vi "Get Param Info.vi"(8 "error in (no error)":errorcluster, 11 "paramID":i32) -> (0 "error out":errorcluster, 1 "paramMin out":dbl, 2 "paramReadOnly out":i32, 3 "function return":i32, 4 "paramMax out":dbl, 5 "paramAvailable out":i32, 6 "paramDefault out":dbl, 7 "paramType out":i32)   [LabVIEW 2020, in "MPH16.lvlib"]
doc: "long GetParamInfo(const long paramID, long &paramType, long &paramAvailable, long &paramReadOnly, double &paramMin, double &paramMax, double &paramDefault);"
uses:
  MPH16.lvlib
  ThorPinholeStepper.dll
panel:
  in  "paramDefault":dbl
  in  "paramMax":dbl
  in  "paramMin":dbl
  in  "paramReadOnly":i32
  in  "paramAvailable":i32
  in  "paramType":i32
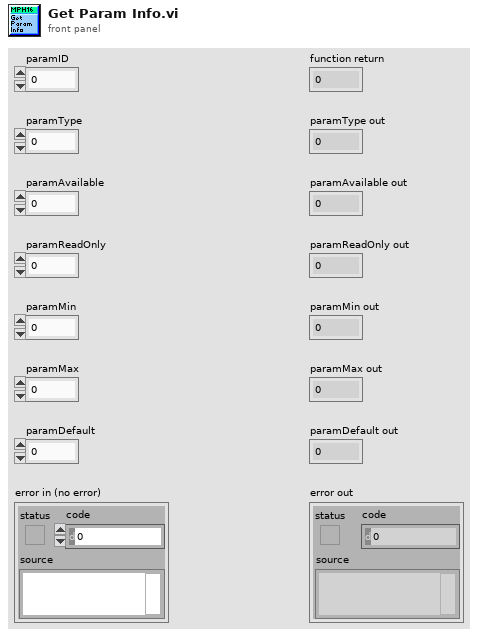
[diagram p1: front panel]
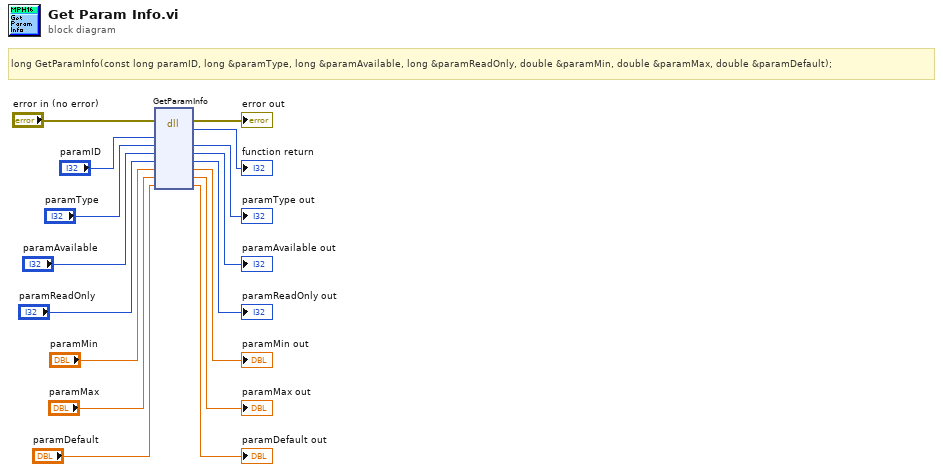
[diagram p0: block diagram]
diagram:
  # "long GetParamInfo(const long paramID, long &paramType, long &paramAvailable, long &paramReadOnly, double &paramMin, double &paramMax, double &paramDefault);"
  n1 = dll-call lib="D:/software/TweezerTron Project/Instruments/Thorlabs/MPH_SDK/ThorPinholeStepper.*" fn="GetParamInfo"(error in="error in (no error)", "paramID"="paramID", "paramType"="paramType", "paramAvailable"="paramAvailable", "paramReadOnly"="paramReadOnly", "paramMin"="paramMin", "paramMax"="paramMax", "paramDefault"="paramDefault") -> (error out=→"error out":errorcluster, →"function return":i32, "paramType"=→"paramType out":i32, "paramAvailable"=→"paramAvailable out":i32, "paramReadOnly"=→"paramReadOnly out":i32, "paramMin"=→"paramMin out":dbl, "paramMax"=→"paramMax out":dbl, "paramDefault"=→"paramDefault out":dbl)  [unwired: 3 in, 1 out]
